vi "Send Error to LabVIEW app.vi"(7 "Server Alias":string, 8 "error in (no error)":errorcluster) -> (0 "error out":errorcluster)   [LabVIEW 2013, in "TS.lvlib"]
doc: "This VI uses the callback VI in order to keep the TS.lvlib separate. We send an error to the LV side. This VI is guaranteed not to output an error."
uses:
  TS.lvlib
  LabVIEW Python Connector Message.ctl
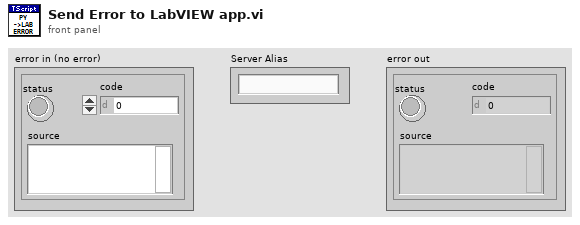
[diagram p1: front panel]
types:
  T1 = typedef "TS.lvlib/LabVIEW Python Connector Message.ctl" = cluster{"Command":string, "Data":string[], "Script ID":i64, "LabVIEW Server ID":string, "Python Message ID":i32}
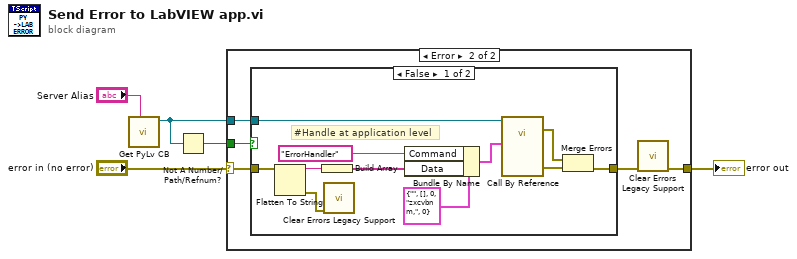
[diagram p0: block diagram]
diagram:
  n1 = call "Get PyLv CB.vi"("Server Alias"="Server Alias") -> ("VI Refnum"=w2:refnum<vi>)  [unwired: 9 in, 1 out]
  n2 = Not A Number/Path/Refnum?(number/path/refnum=w2) -> (NaN/Path/Refnum?=w4:bool)
  n3 = case shown="Error" "error in (no error)" {
    selector: "error in (no error)" -> [w6 w8]
    tunnel: [w6 w7] -> w5
    tunnel: w4 -> [_ w10]
    tunnel: w2 -> [_ w9]
    frame No Error {
    }
    frame Error {
      n4 = case shown="False" w10 {
        tunnel: w8 -> [w19 w23]
        tunnel: [w22 w23] -> w11
        tunnel: w9 -> [w15 _]
        frame False {
          # "#Handle at application level"
          n5 = Flatten To String(anything=w19) -> (data string=w18:string, error out=w16:errorcluster)  [unwired: 3 in, 1 out]
          n6 = Build Array(w18) -> (w17:string[])
          n7 = call "Clear Errors Legacy Support.vi"("error in (no error)"=w16) -> ()  [unwired: 5 in, 2 out]
          n8 = Bundle By Name(cluster=T1 {"Command"="", "Data"=[], "Script ID"=0, "LabVIEW Server ID"="zxcvbnm,", "Python Message ID"=0} ("Message to LabVIEW App"), "Command"="ErrorHandler", "Data"=w17) -> (w14:T1)
          n9 = call-by-ref "?"(reference=w15, "Message to LabVIEW App"=w14) -> (error out=w12:errorcluster, 0:"error out"=w13:errorcluster)  [unwired: 11 in, 1 out]
          n10 = Merge Errors(w12, w13) -> (w22:errorcluster)
        }
        frame True {
          # "Not a valid reference\nNo op"
        }
      }
      n11 = call "Clear Errors Legacy Support.vi"("error in (no error)"=w11) -> ("error out"=w7:errorcluster)  [unwired: 5 in, 1 out]
    }
  }
  "error out" <- w5
